vi "XY Graph Denoise Multiple Plots.vi"(7 "Wavelet Analysis Options":T1={"Wavelet"=enum."db02", "Option for Approximate Coefficients"=enum."None", "# Levels"=1, "Threshold Settings"={"Thresholding Rule"=enum."Universal", "Rescaling Method"=enum."Single level", "Soft Threshold?"=TRUE}, "Wavelet Transform Type"=enum."Discrete"}, 8 "error in (no error)":errorcluster, 10 "Selected Plots":i32[](array[numeric]), 11 "Selected Plot Info":T2) -> (0 "error out":errorcluster, 1 "Denoised Plot Message":string, 3 "Last Denoised Plot":cluster{"t Array":dbl[], "IRF Array":dbl[]}, 4 "Single Plot?":bool)   [LabVIEW 2021, in "XY Graph Add-Ons.lvlib"]
uses:
  XY Graph Add-Ons.lvlib
  XY Graph Selected Plot Info.ctl
  XY Graph Refnum.ctl
  <vilib>/Utility/miscctls.llb/LVPoint32TypeDef.ctl
  Math/Advanced Signal Processing Toolkit/Wavelet Analysis Options.ctl
  Strings/Strings.lvlib
  Math/Math.lvlib
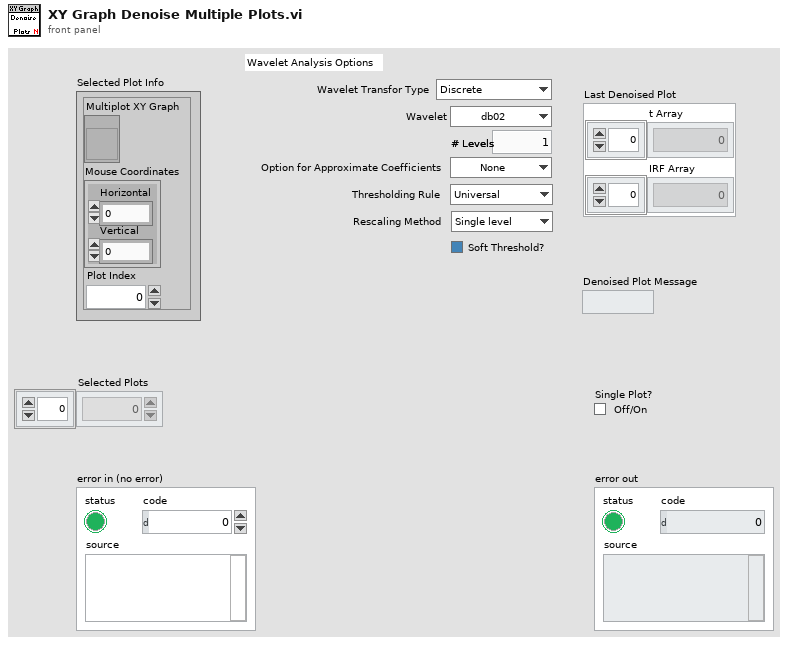
[diagram p1: front panel]
types:
  T1 = typedef "Math.lvlib/Wavelet Analysis Options.ctl" = cluster{"Wavelet":enum16{"db02", "db03", "db04", "db05", "db06", "db07", "db08", "db09", "db10", "db11", "db12", "db13", "db14", "Haar", "bior1_3", "bior1_5", "bior2_2", "bior2_4", "bior2_6", "bior2_8", "bior3_1", "bior3_3", "bior3_5", "bior3_7", "bior3_9", "bior4_4 (FBI)", "bior5_5", "bior6_8", "coif1", "coif2", "coif3", "coif4", "coif5", "sym2", "sym3", "sym4", "sym5", "sym6", "sym7", "sym8"}, "Option for Approximate Coefficients":enum16{"None", "Threshold", "Detrend"}, "# Levels":i32, "Threshold Settings":cluster{"Thresholding Rule":enum16{"SURE", "Hybrid", "Universal", "Minimax"}, "Rescaling Method":enum16{"One", "Single level", "Multiple levels"}, "Soft Threshold?":bool}, "Wavelet Transform Type":enum16{"Discrete", "Undecimated"}}
  T2 = typedef "XY Graph Add-Ons.lvlib/XY Graph Selected Plot Info.ctl" = cluster{"Multiplot XY Graph":T3, "Mouse Coordinates":T4, "Plot Index":i32}
  T3 = typedef "XY Graph Add-Ons.lvlib/XY Graph Refnum.ctl" = refnum<vi>
  T4 = typedef "LVPoint32TypeDef.ctl" = cluster{"Horizontal":i32, "Vertical":i32}
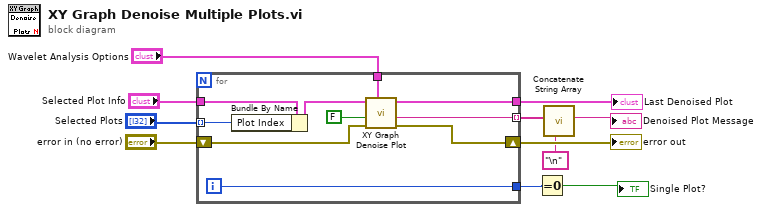
[diagram p0: block diagram]
diagram:
  n1 = for {
    tunnel: "Selected Plot Info" -> [w21]
    tunnel: [w19] -> w6 mode=indexing
    tunnel: [w17] -> w8
    shift-right: [w18] -> w9
    shift-left: "error in (no error)" -> [w20]
    tunnel: "Selected Plots" -> [w15] mode=indexing
    tunnel: [w14] -> w3
    tunnel: "Wavelet Analysis Options" -> [w12]
    i -> [w14]
    n2 = Bundle By Name(cluster=w21, "Plot Index"=w15) -> (w16:T2)
    n3 = call "XY Graph Denoise Plot.vi"("Wavelet Analysis Options"=w12, "error in (no error)"=w20, "Replace Plot (T)?"=FALSE, "Selected Plot Info"=w16) -> ("Error Out"=w18:errorcluster, "Message"=w19:string, "Denoised Plot"=w17:cluster{"t Array":dbl[], "IRF Array":dbl[]})  [unwired: 5 in]
  }
  "error out" <- w9
  "Last Denoised Plot" <- w8
  n4 = Equal To 0?(x=w3) -> (x = 0?=→"Single Plot?":bool)
  n5 = call "Concatenate String Array.vi"("Separator (TAB)"="\n", "String Array"=w6) -> ("Formatted String"=→"Denoised Plot Message":string)  [unwired: 9 in]
